vi "Launcher.vi"() -> ()   [LabVIEW 2022 SP3]
uses:
  Phoenix/Phoenix.lvclass
  Phoenix/UI.vi
panel:
  in  "vi path":path
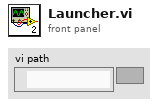
[diagram p1: front panel]
types:
  T1 = enum32{"Invalid", "Standard", "Closed", "Hidden", "Minimized", "Maximized"}
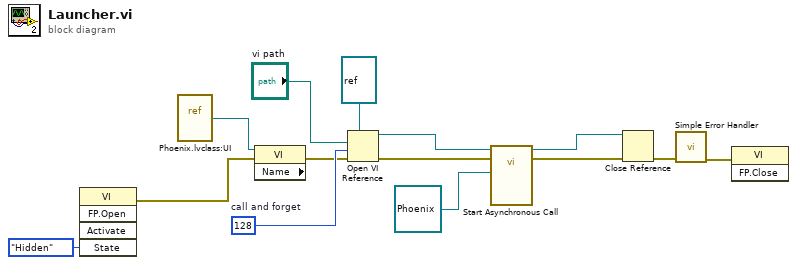
[diagram p0: block diagram]
diagram:
  w13 = 128  # call and forget
  n1 = invoke class="VI" method="FP.Open"("State"=T1."Hidden") -> (error out=w4:errorcluster)  [unwired: 4 in, 4 out]
  n2 = vi-ref "Phoenix.lvclass:UI.vi"() -> (w2:refnum<vi>)
  n3 = property class="VI" props=["Name"](reference=w2, error in=w4) -> (error out=w6:errorcluster)  [unwired: 2 out]
  n4 = Open VI Reference(type specifier VI Refnum (for type only)=refnum<vi> refnum, vi path="vi path", options=w13, error in (no error)=w6) -> (vi reference=w11:refnum<vi>, error out=w10:errorcluster)  [unwired: 2 in]
  n5 = call-by-ref "Start Asynchronous Call"(reference=w11, error in=w10, "Phoenix in"=refnum<class "Phoenix.lvclass"> refnum) -> (reference out=w8:refnum<vi>, error out=w9:errorcluster)  [unwired: 9 in, 2 out]
  n6 = Close Reference(reference=w8, error in (no error)=w9) -> (error out=w7:errorcluster)
  n7 = call <vilib>:"Simple Error Handler.vi"("error in (no error)"=w7) -> ("error out"=w3:errorcluster)  [unwired: 4 in, 4 out]
  n8 = invoke class="VI" method="FP.Close"(error in=w3) -> ()  [unwired: 2 in, 3 out]
